vi "Set Inspect Speed.vi"(11 "Inspect Speed":u16) -> ()   [LabVIEW 2015, in "Tool Cfg.lvlib"]
uses:
  Tool Cfg.lvlib
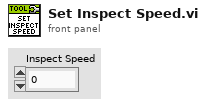
[diagram p1: front panel]
types:
  T1 = typedef "Tool Cfg.lvlib/_Motor Block Cluster_v2--typedef.ctl" = cluster{"MinMotor Speed":u16, "MaxMotor Speed":u16, "Homing Speed":u16, "Jog Speed":u16, "Inspect Speed":u16, "VBlk Speed":u16, "CleaningPos":i32, "Safe Zone":i32, "Has Motor":bool, "Use Home Index":bool}
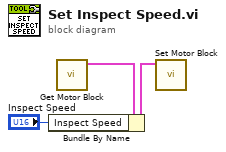
[diagram p0: block diagram]
diagram:
  n1 = call "Get Motor Block.vi"() -> ("Motor Block"=w3:T1)  [unwired: 11 in]
  n2 = Bundle By Name(cluster=w3, "Inspect Speed"="Inspect Speed") -> (w1:T1)
  n3 = call "Set Motor Block.vi"("Motor Block"=w1) -> ()  [unwired: 11 in]
